vi "Write Parameters CCD modes.vi"(8 "error in (no error)":errorcluster, 10 "Parameters CCD modes":T1={"Image \nInitial Line"=0, "Image\nInitial Column"=0, "Image\nFinal Line"=0, "Image\nFInal Column"=0, "Vertical\nBinning"=0, "Horizontal\nBinning"=0, "Pre-amplification\nGain"=0, "CCD\nEM Gain"=2, "Readout\nRate"=0, "Shutter\nOpenning Time"=1, "Shutter\nClosing Time"=1, "Vertical\nShift Speed"=0, "Read\nMode"=0, "Vertical\nClock Voltage"=0, "A/D \nChannel"=0, "Shutter\nMode"=0, "Shutter\nTTL"=0, "Trigger\nMode"=0, "Frame\nTransfer"=FALSE, "Acquisition\nMode"=0, "CCD \nEM Mode"=0} caption="Preview Configuration for all channels:" {"CCD \nEM Mode" items=["Electron Mult.", "Conventional"]; "Acquisition\nMode" items=["None", "Single Scan", "Accumulate", "Kinectics", "Fast Kinectics", "None2", "Frame Transfer", "None3", "None4", "Time Delayed Integration"]; "Trigger\nMode" items=["Internal"=0, "Ext. Start"=6]; "Shutter\nTTL" items=["High", "Low"]; "Shutter\nMode" items=["Open"=1, "Closed"=2]; "Vertical\nClock Voltage" items=["Normal", "+1", "+2", "+3", "+4"]; "Read\nMode" items=["Full-Vertical-Binning", "Multi-Track", "Random-Track", "Single-Track", "Image"]; "Vertical\nShift Speed" items=["0.6", "1.13", "2.2", "4.33"]; "Shutter\nClosing Time" min=1; "Shutter\nOpenning Time" min=1; "Readout\nRate" items=["1 MHz", "0.1 MHz"]; "CCD\nEM Gain" min=2 max=300 step=1; "Pre-amplification\nGain" items=["Gain 1", "Gain 2"]}, 11 "S4GUI in":refnum<class "S4GUI.lvclass">) -> (0 "error out":errorcluster, 3 "S4GUI out":refnum<class "S4GUI.lvclass">)   [LabVIEW 2018, in "S4GUI.lvclass"]
uses:
  S4GUI.lvclass
  S4GUI.lvclass/S4GUI.ctl
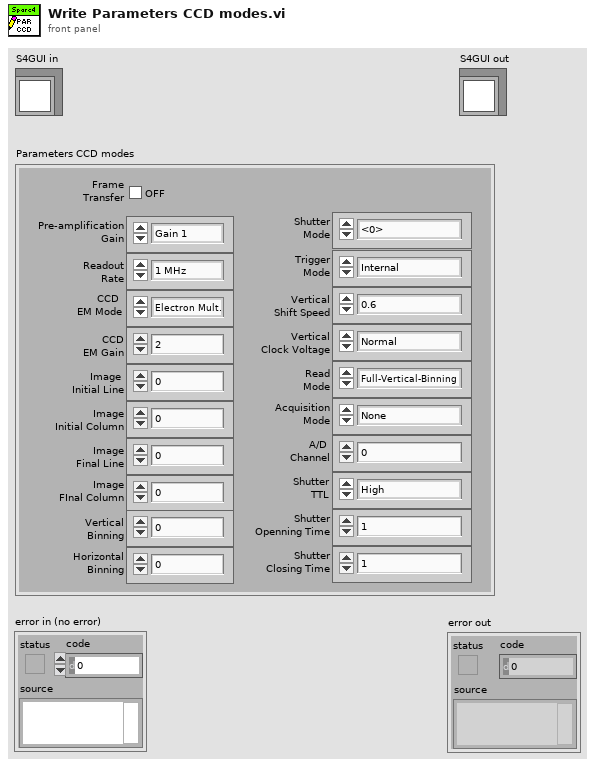
[diagram p1: front panel]
types:
  T1 = cluster{"Image \nInitial Line":u16, "Image\nInitial Column":u16, "Image\nFinal Line":u16, "Image\nFInal Column":u16, "Vertical\nBinning":u16, "Horizontal\nBinning":u16, "Pre-amplification\nGain":u8, "CCD\nEM Gain":u16, "Readout\nRate":u8, "Shutter\nOpenning Time":i32, "Shutter\nClosing Time":i32, "Vertical\nShift Speed":u8, "Read\nMode":u8, "Vertical\nClock Voltage":u8, "A/D \nChannel":u32, "Shutter\nMode":u16, "Shutter\nTTL":u16, "Trigger\nMode":u16, "Frame\nTransfer":bool, "Acquisition\nMode":u8, "CCD \nEM Mode":u8}
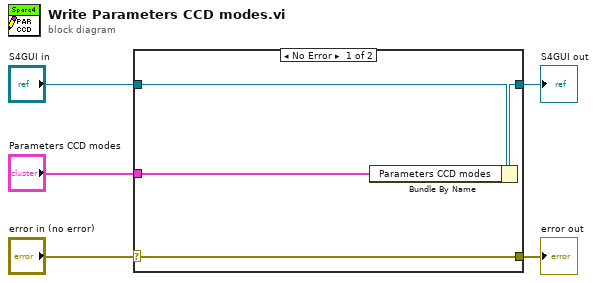
[diagram p0: block diagram]
diagram:
  n1 = case shown="No Error" "error in (no error)" {
    selector: "error in (no error)" -> [w9 w10]
    tunnel: [w9 w10] -> w4
    tunnel: [w7 w11] -> w2
    tunnel: "S4GUI in" -> [w8 w11]
    tunnel: "Parameters CCD modes" -> [w6 _]
    frame No Error {
      n2 = Bundle By Name(cluster=w8, "Parameters CCD modes"=w6) -> (w7:refnum<class "S4GUI.lvclass">)
    }
    frame Error {
    }
  }
  "error out" <- w4
  "S4GUI out" <- w2
